vi "About Program.vi"(1 "Diplay Text In":string) -> ()   [LabVIEW 2021]
panel:
  out "Diplay Text":string
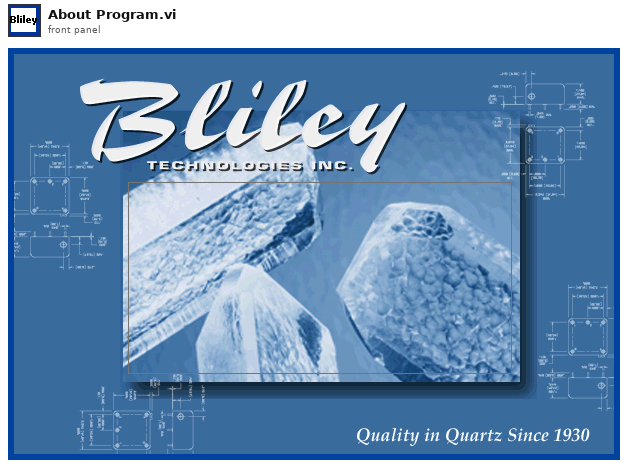
[diagram p1: front panel]
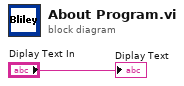
[diagram p0: block diagram]
diagram:
  "Diplay Text" <- "Diplay Text In"
